vi "MeasureAtFreq.vi"(8 "error in (no error)":errorcluster, 10 "Frequency (Hz)":dbl, 11 "SpecA_ESA in":refnum<class "SpecA_ESA.lvclass">) -> (0 "error out":errorcluster, 2 "Power (dBm)":dbl, 3 "SpecA_ESA out":refnum<class "SpecA_ESA.lvclass">)   [LabVIEW 2014, in "SpecA_ESA.lvclass"]
uses:
  SpecA_ESA.lvclass
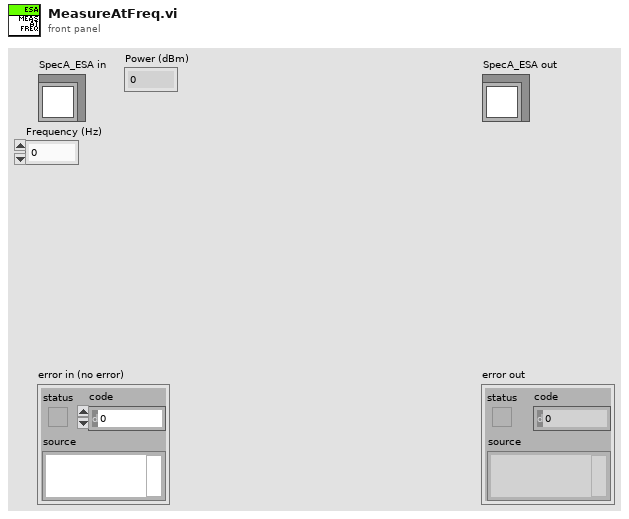
[diagram p1: front panel]
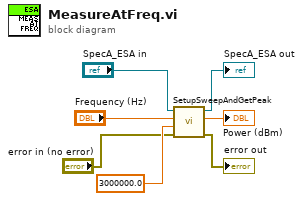
[diagram p0: block diagram]
diagram:
  n1 = call-dynamic "SetupSweepAndGetPeak.vi"("error in (no error)"="error in (no error)", "Span(Hz)"=3000000.0, "Center Frequency(Hz)"="Frequency (Hz)", "SpecA_ESA in"="SpecA_ESA in") -> ("error out"=→"error out":errorcluster, "Calibrated Amplitude (dBm)"=→"Power (dBm)":dbl, "SpecA_ESA out"=→"SpecA_ESA out":refnum<class "SpecA_ESA.lvclass">)  [unwired: 4 in, 1 out]
